vi "configure.vi"(8 "error in (no error)":errorcluster, 11 "GenericPlugin in":refnum<class "TrajectoryMH100122AODRAPS.lvclass">) -> (0 "error out":errorcluster, 3 "GenericPlugin out":refnum<class "TrajectoryMH100122AODRAPS.lvclass">)   [LabVIEW 2010, in "TrajectoryMH100122AODRAPS.lvclass"]
doc: "The dynamic dispatch version of this VI loads and displays the configuration file associated with the plug-in object. The user modify and save the configuration data."
uses:
  TrajectoryMH100122AODRAPS.lvclass
  common/xcontrols/XComponentSpecification/XComponentSpecification/XComponentSpecification.xctl
  TrajectoryMH100122AODRAPS.lvclass/TrajectoryMH100122AODRAPS.ctl
  common/classes/GenericComponent/GenericComponent/GenericComponent.lvclass
panel:
  in  "FPGA Wrapper path":T1(xcontrol)
  in  "ROI color":u32(colorbox)=6618880
  in  "motion correction array size":u8=1 min=1
  in  "XML path zoom":string="Image/StructuredAnnotations/XmlStringAnnotation/HelioScan/ScanHead/settings/"
  in  "cancel":bool
  in  "save":bool
  out "Configuration name":string
  # "Configure TrajectoryAODRAPS"
  # "The TrajectoryMH100122AODRAPS component controls the random access pattern scanning trajectory for the FPGA. \n\nEach FPGA controls the home built direct digital synthesizer (DDS) board that synthesizes the wave forms for the acousto-optic deflectors (AOD)."
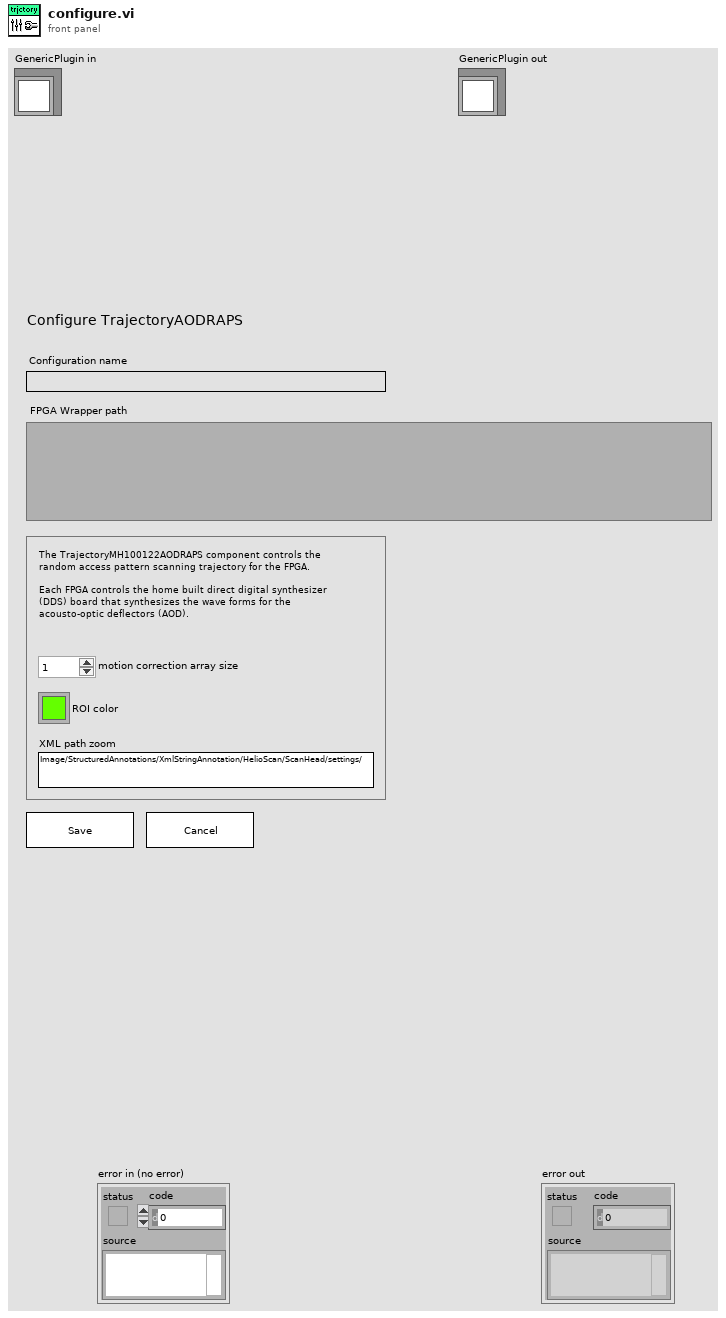
[diagram p1: front panel]
types:
  T1 = cluster{"class path":string, "configuration":string, "label":string, "settings name":string}
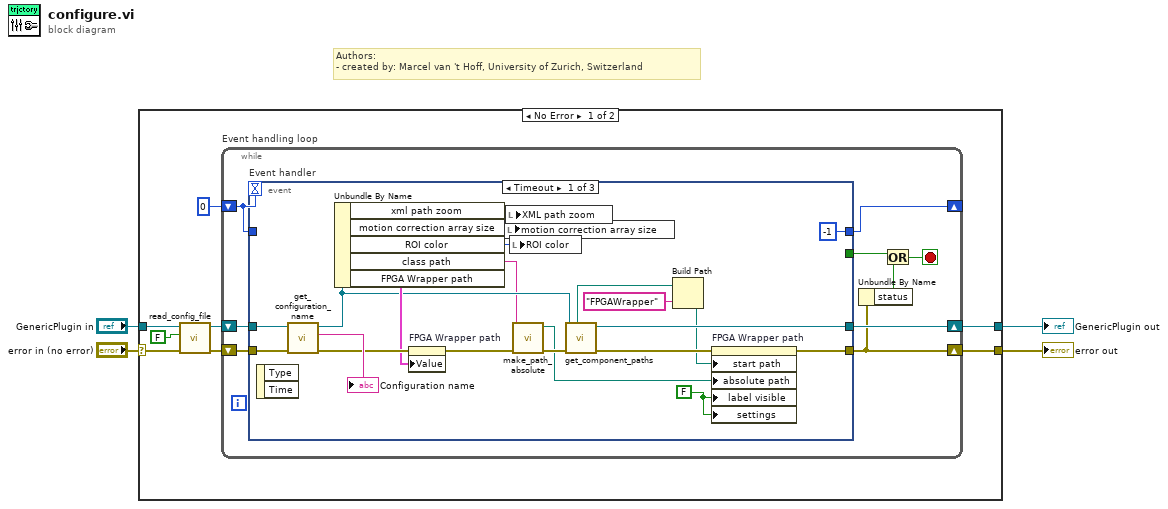
[diagram p0: block diagram]
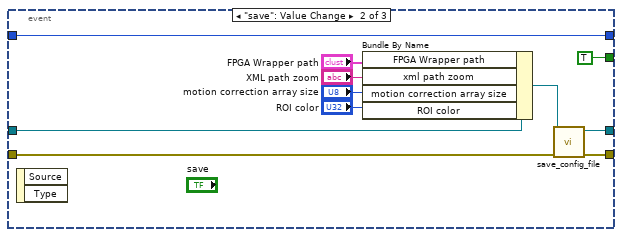
[diagram p2: hidden frame]
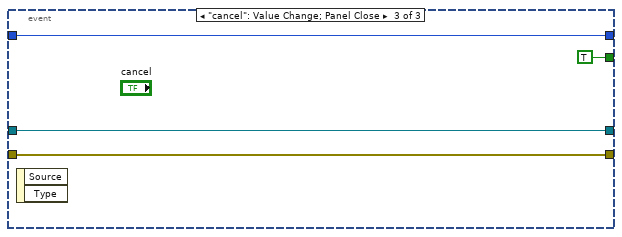
[diagram p3: hidden frame]
diagram:
  # "Authors: \n- created by: Marcel van 't Hoff, University of Zurich, Switzerland"
  n1 = case shown="No Error" "error in (no error)" {
    selector: "error in (no error)" -> [w9 w59]
    tunnel: [w11 w59] -> w4
    tunnel: [w10 w58] -> w3
    tunnel: "GenericPlugin in" -> [w8 w58]
    frame No Error {
      n2 = call-dynamic "read_config_file.vi"("error in (no error)"=w9, "force load?"=FALSE, "GenericPlugin in"=w8) -> ("error out"=w5:errorcluster, "GenericPlugin out"=w7:refnum<class "TrajectoryMH100122AODRAPS.lvclass">)  [unwired: 7 out]
      n3 = while "Event handling loop" {
        shift-right: [w19] -> _
        shift-left: 0 -> [w20]
        shift-right: [w16] -> w11
        shift-left: w5 -> [w21]
        shift-right: [w17] -> w10
        shift-left: w7 -> [w18]
        stop <- w14 stop-if-true
        n4 = event "Event handler" shown="[0] Timeout" {
          selector: _ -> [_ _ _]
          dyn-events: _ -> [_ _ _]
          timeout: w20 -> [_ _ _]
          tunnel: w21 -> [w41 w52 w56]
          tunnel: [-1 w53 w57] -> w19
          tunnel: w20 -> [_ w53 w57]
          tunnel: [w28 w51 w56] -> w16
          tunnel: [_ TRUE TRUE] -> w13
          tunnel: w18 -> [w40 w48 w54]
          tunnel: [w24 w50 w54] -> w17
          event Timeout {
            w22 = FALSE ("label visible")
            n5 = event-data() -> ()  [unwired: 3 out]
            n6 = call "get_configuration_name.vi"("error in (no error)"=w41, "GenericPlugin.lvclass in"=w40) -> ("error out"=w35:errorcluster, "configuration name"=→"Configuration name":string, "GenericPlugin.lvclass out"=w27:refnum<class "TrajectoryMH100122AODRAPS.lvclass">)  [unwired: 7 in]
            n7 = Unbundle By Name(w27) -> ("xml path zoom"=w37:string, "motion correction array size"=w38:u8, "ROI color"=w36:u32, "class path"=w26:string, "FPGA Wrapper path"=w34:T1)
            n8 = property on="FPGA Wrapper path" class="XComponentSpecification (strict"(error in=w35, "Value"=w34) -> (error out=w31:errorcluster)  [unwired: 1 in, 1 out]
            n9 = local write "motion correction array size"(w38) -> ()
            n10 = local write "XML path zoom"(w37) -> ()
            n11 = local write "ROI color"(w36) -> ()
            n12 = call "make_path_absolute.vi"("error in (no error)"=w31, "relative path"=w26) -> ("error out"=w30:errorcluster, "absolute path"=w25:path)  [unwired: 8 in]
            n13 = call-dynamic "get_component_paths.vi"("error in (no error)"=w30, "GenericComponent in"=w27) -> ("error out"=w29:errorcluster, "GenericComponent out"=w24:refnum<class "TrajectoryMH100122AODRAPS.lvclass">, "components directory"=w32:path)  [unwired: 4 in, 3 out]
            n14 = Build Path(base path=w32, name or relative path="FPGAWrapper") -> (appended path=w23:path)
            n15 = property on="FPGA Wrapper path" class="XComponentSpecification (strict"(error in=w29, "start path"=w23, "absolute path"=w25, "label visible"=w22, "settings"=w22) -> (error out=w28:errorcluster)  [unwired: 1 in, 1 out]
          }
          event "save": Value Change {
            n16 = event-data() -> ()  [unwired: 3 out]
            n17 = Bundle By Name(cluster=w48, "FPGA Wrapper path"="FPGA Wrapper path", "xml path zoom"="XML path zoom", "motion correction array size"="motion correction array size", "ROI color"="ROI color") -> (w47:refnum<class "TrajectoryMH100122AODRAPS.lvclass">)
            n18 = call-dynamic "save_config_file.vi"("error in (no error)"=w52, "GenericPlugin in"=w47) -> ("error out"=w51:errorcluster, "GenericPlugin out"=w50:refnum<class "TrajectoryMH100122AODRAPS.lvclass">)  [unwired: 2 in, 6 out]
          }
          event "cancel": Value Change; Panel Close {
            n19 = event-data() -> ()  [unwired: 3 out]
          }
        }
        n20 = Unbundle By Name(w16) -> ("status"=w15:bool)
        n21 = Or(x=w13, y=w15) -> (x .or. y?=w14:bool)
      }
    }
    frame Error {
    }
  }
  "error out" <- w4
  "GenericPlugin out" <- w3
